vi "Select Filter Structure.vi"(10 "filter structure option":T1=2 items=["IIR 2nd Order", "IIR 4th Order", "Auto Select"], 11 "filter type":T2) -> (3 "filter structure":enum32{"IIR 2nd Order", "IIR 4th Order"}(ring))   [LabVIEW 2020, in "NI_AALBase.lvlib"]
uses:
  <vilib>/Analysis/NI_AALBase.lvlib
  <vilib>/Analysis/3filter.llb/Filter Passband Type.ctl
  <vilib>/Analysis/3filter.llb/Filter Structure Type.ctl
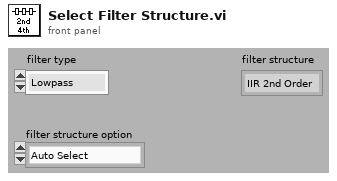
[diagram p1: front panel]
types:
  T1 = typedef "NI_AALBase.lvlib/Filter Structure Type.ctl" = u16
  T2 = typedef "NI_AALBase.lvlib/Filter Passband Type.ctl" = enum32{"Lowpass", "Highpass", "Bandpass", "Bandstop"}
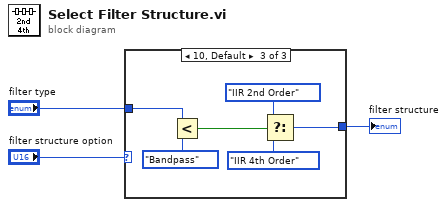
[diagram p0: block diagram]
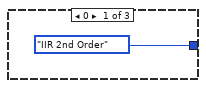
[diagram p2: hidden frame]
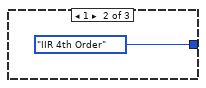
[diagram p3: hidden frame]
diagram:
  n1 = case shown="10, Default" "filter structure option" {
    tunnel: [enum32{"IIR 2nd Order", "IIR 4th Order"}."IIR 2nd Order" ("filter structure") enum32{"IIR 2nd Order", "IIR 4th Order"}."IIR 4th Order" ("filter structure") w7] -> w2
    tunnel: "filter type" -> [_ _ w11]
    frame 0 {
    }
    frame 1 {
    }
    frame 10, Default {
      n2 = Less?(x=w11, y=Filter_Passband_Type."Bandpass") -> (x < y?=w9:bool)
      n3 = Select(t=enum32{"IIR 2nd Order", "IIR 4th Order"}."IIR 2nd Order" ("filter structure"), s=w9, f=enum32{"IIR 2nd Order", "IIR 4th Order"}."IIR 4th Order" ("filter structure")) -> (s? t:f=w7:enum32{"IIR 2nd Order", "IIR 4th Order"})
    }
  }
  "filter structure" <- w2
